vi "Rhythm Pattern Test.vi"() -> ()   [LabVIEW 2020]
uses:
  Rhythm Pattern VIs/Rhythm-Properties.ctl
  Rhythm Pattern VIs/Rhythm-Data.ctl
panel:
  out "Y-axis":dbl(slide) scale=-0.5..5.5
  out "Pattern":cluster{"X":dbl, "Y":dbl}[](graph)
  in  "Save Button":bool
  out "exit signal":bool
  out "Graph":dbl[](graph)
  out "finished":errorcluster
  in  "Play Button":bool
  in  "Refresh Button":bool
  in  "Quit Button":bool
  in  "Frame size (s)":dbl=0.25
  in  "Sampling rate (Hz)":dbl=50000.0
  in  "Properties":T1={"Method"=enum."Interval", "Waveform"=enum."Noise", "Time"={"Ramp (ms)"=5.0, "Duration (ms)"=25.0, "Interval (ms)"=400.0}, "Expr"="50:50:300", "Pattern"={"# rand"=5.0, "reg fraction"=1.0, "Rcyc"=5, "pattern"=enum."RAND-REG", "Lsignal (cyc)"={"Min"=12, "Max"=12}, "Trans (cyc)"={"Min"=4, "Max"=5}}}
  in  "Stop Button":bool
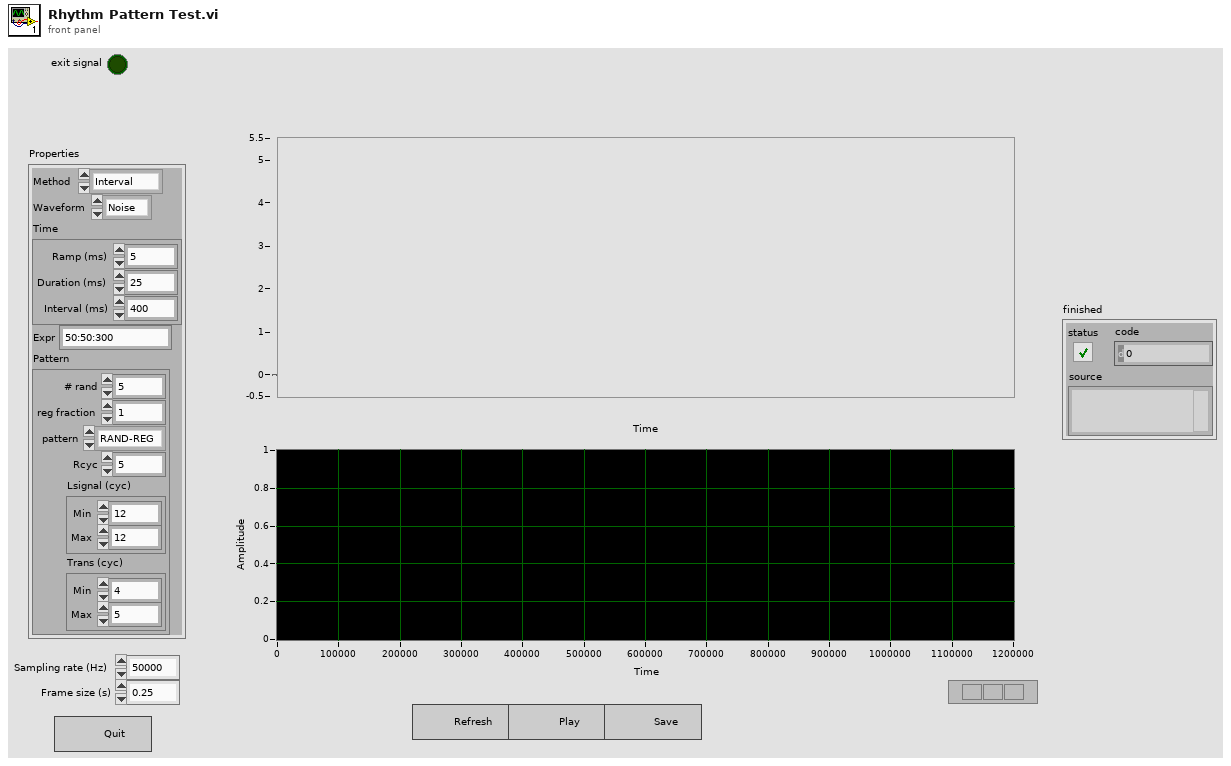
[diagram p1: front panel]
types:
  T1 = typedef "Rhythm-Properties.ctl" = cluster{"Method":enum16{"Telegraph", "Interval"}, "Waveform":enum16{"Click", "Noise"}, "Time":cluster{"Ramp (ms)":dbl, "Duration (ms)":dbl, "Interval (ms)":dbl}, "Expr":string, "Pattern":cluster{"# rand":dbl, "reg fraction":dbl, "Rcyc":i32, "pattern":enum16{"RAND-REG", "REG-RAND", "RAND", "REG", "STEP", "CF"}, "Lsignal (cyc)":cluster{"Min":i32, "Max":i32}, "Trans (cyc)":cluster{"Min":i32, "Max":i32}}}
  T2 = typedef "Rhythm-Data.ctl" = cluster{"Values":dbl[], "Gate":dbl[], "Rep":i32, "PhaseIndex":i32, "transition":i32, "nrepeat":i32, "Method":enum16{"Telegraph", "Interval"}, "Fs":dbl, "Time":cluster{"Ramp (ms)":dbl, "Duration (ms)":dbl, "Interval (ms)":dbl}, "Waveform":enum16{"Click", "Noise"}}
  T3 = cluster{"Data":T2, "Sampling rate (Hz)":dbl, i32, "#frames":i32}
  T4 = enum8{"Enabled", "Disabled", "Disabled and Grayed Out"}
  T5 = typedef "Sound Output Task ID.ctl" = u32
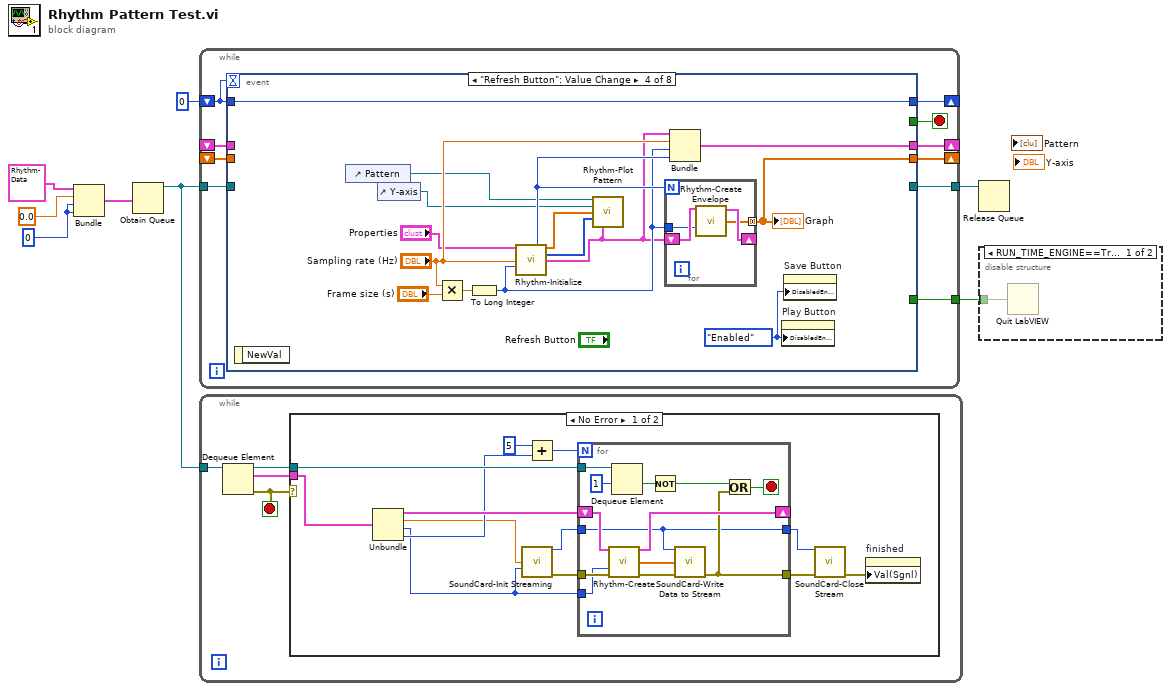
[diagram p0: block diagram]
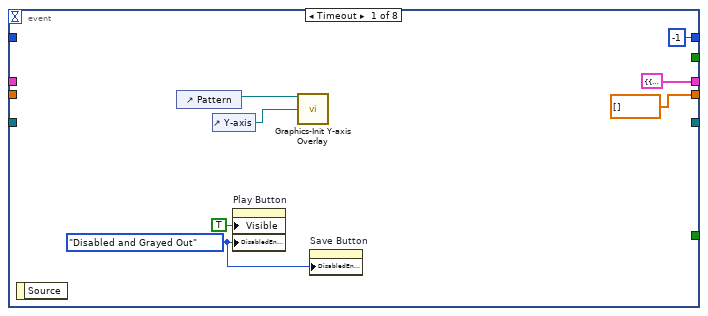
[diagram p4: hidden frame]
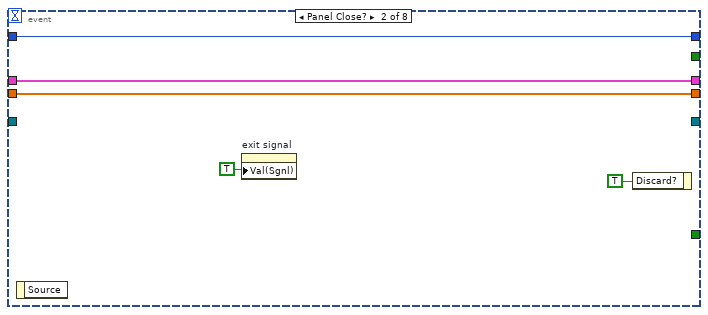
[diagram p5: hidden frame]
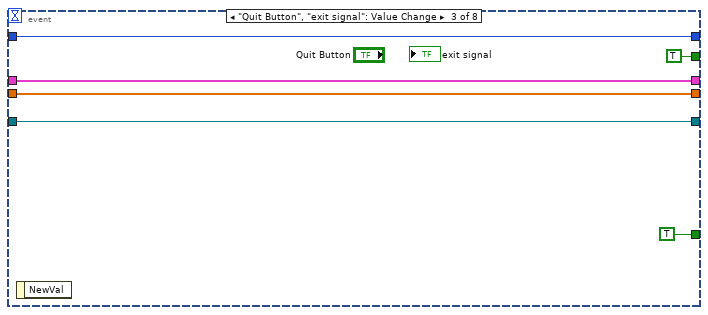
[diagram p6: hidden frame]
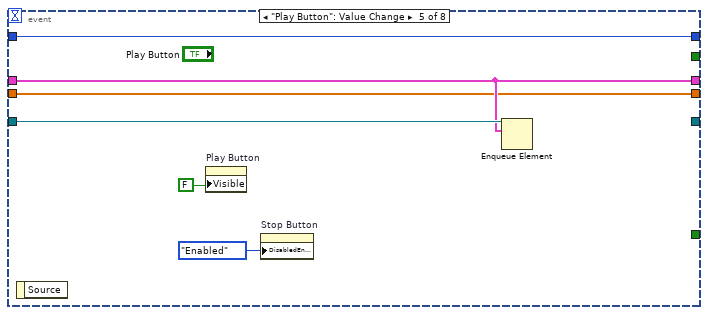
[diagram p7: hidden frame]
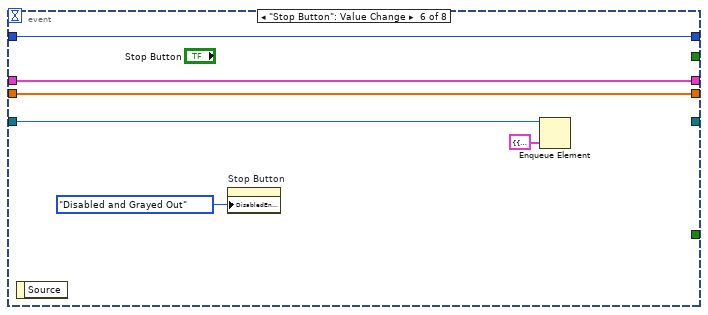
[diagram p8: hidden frame]
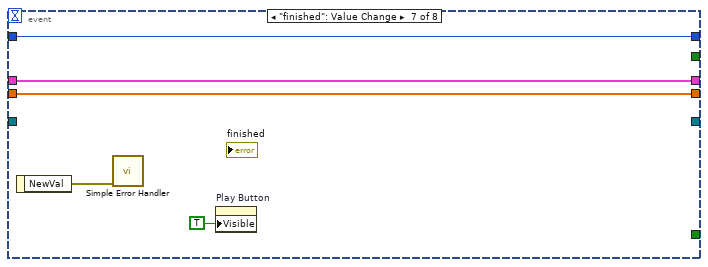
[diagram p9: hidden frame]
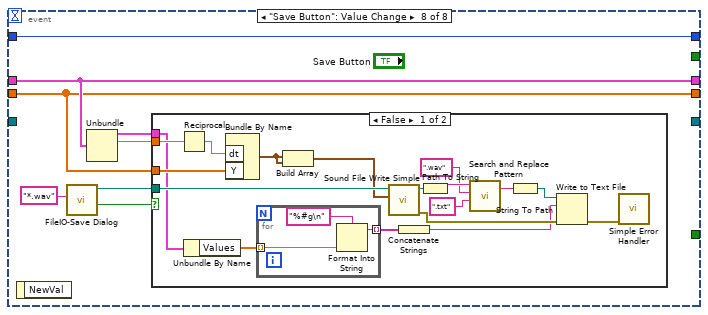
[diagram p10: hidden frame]
diagram:
  w2 = 0
  n1 = Bundle("Data"=T2 {"Values"=array[5000 elements], "Gate"=[8.0], "Rep"=0, "PhaseIndex"=5000, "transition"=0, "nrepeat"=0, "Method"=enum."Telegraph", "Fs"=0.0, "Time"={"Ramp (ms)"=0.0, "Duration (ms)"=0.0, "Interval (ms)"=0.0}, "Waveform"=enum."Click"}, 0.0, w2, w2) -> (w5:cluster{"Data":T2, dbl, i32, i32})  [unwired: 1 in]
  n2 = Obtain Queue(element data type=w5) -> (queue out=w6:refnum<queue>)  [unwired: 4 in, 2 out]
  n3 = while {
    shift-right: [w16] -> _
    shift-left: 0 -> [w17]
    tunnel: w6 -> [w15]
    tunnel: [w14] -> w7
    tunnel: [w13] -> w1
    shift-right: [w12] -> _
    shift-left: _ -> [w11]
    shift-right: [w10] -> _
    shift-left: _ -> [w9]
    stop <- w18 stop-if-true
    n4 = event shown="[3] \"Refresh Button\": Value Change" {
      selector: _ -> [_ _ _ _ _ _ _ _]
      dyn-events: _ -> [_ _ _ _ _ _ _ _]
      timeout: w17 -> [_ _ _ _ _ _ _ _]
      tunnel: [_ _ TRUE _ _ _ _ _] -> w18
      tunnel: w17 -> [_ w30 w35 w51 w61 w67 w72 w80]
      tunnel: [-1 w30 w35 w51 w61 w67 w72 w80] -> w16
      tunnel: w15 -> [_ _ w34 _ w58 w66 _ _]
      tunnel: [_ _ w34 _ _ _ _ _] -> w14
      tunnel: [_ _ TRUE _ _ _ _ _] -> w13
      tunnel: [T3 {"Data"={"Values"=[], "Gate"=[], "Rep"=0, "PhaseIndex"=0, "transition"=0, "nrepeat"=0, "Method"=enum."Telegraph", "Fs"=0.0, "Time"={"Ramp (ms)"=0.0, "Duration (ms)"=0.0, "Interval (ms)"=0.0}, "Waveform"=enum."Click"}, "Sampling rate (Hz)"=0.0, 0, "#frames"=0} w27 w32 w45 w57 w64 w69 w76] -> w12
      tunnel: w11 -> [_ w27 w32 _ w57 w64 w69 w76]
      tunnel: [dbl[] [] ("Y") w26 w31 w44 w56 w63 w68 w74] -> w10
      tunnel: w9 -> [_ w26 w31 _ w56 w63 w68 w74]
      event Timeout {
        w23 = T4."Disabled and Grayed Out" ("Disabled")
        n5 = event-data() -> ()  [unwired: 1 in, 1 out]
        n6 = control-ref of="Pattern"() -> (w20:refnum<vi>)
        n7 = control-ref of="Y-axis"() -> (w19:refnum<vi>)
        n8 = property on="Play Button" class="Bool"("Visible"=TRUE, "DisabledEnum"=w23) -> ()  [unwired: 2 in, 2 out]
        n9 = call "Graphics-Init Y-axis Overlay.vi"("Ctl Refnum"=w20, "Y-axis slider"=w19) -> ()  [unwired: 13 in, 1 out]
        n10 = property on="Save Button" class="Bool"("DisabledEnum"=w23) -> ()  [unwired: 2 in, 2 out]
      }
      event Panel Close? {
        n11 = event-data() -> ()  [unwired: 1 in, 1 out]
        n12 = property on="exit signal" class="Bool (strict)"("Val(Sgnl)"=TRUE ("Value (Signaling)")) -> ()  [unwired: 2 in, 2 out]
        n13 = event-data("Discard?"=TRUE) -> ()  [unwired: 1 in, 1 out]
      }
      event "Quit Button", "exit signal": Value Change {
        n14 = event-data() -> ()  [unwired: 1 in, 1 out]
      }
      event "Refresh Button": Value Change {
        w43 = T4."Enabled" ("Disabled")
        n15 = event-data() -> ()  [unwired: 1 in, 1 out]
        n16 = control-ref of="Pattern"() -> (w41:refnum<vi>)
        n17 = control-ref of="Y-axis"() -> (w40:refnum<vi>)
        n18 = Multiply(x="Sampling rate (Hz)", y="Frame size (s)") -> (x*y=w50:dbl)
        n19 = To Long Integer(number=w50) -> (32bit integer=w46:i32)
        n20 = call "Rhythm-Initialize.vi"("Rhythm"="Properties", "Sampling rate (Hz)"="Sampling rate (Hz)", "Npts"=w46) -> ("#frames"=w47:i32, "Values"=w39:dbl[], "Mask"=w38:i32[], "Data"=w37:T2)  [unwired: 8 in, 1 out]
        n21 = call "Rhythm-Plot Pattern.vi"("Graph"=w41, "Y-axis slider"=w40, "Values"=w39, "Mask"=w38, "Data"=w37) -> ()  [unwired: 10 in, 1 out]
        n22 = for {
          N: w47 -> [_]
          tunnel: w46 -> [w52]
          shift-right: [w54] -> _
          shift-left: w37 -> [w55]
          tunnel: [w53] -> w44 mode=concatenating
          n23 = call "Rhythm-Create Envelope.vi"("Data in"=w55, "Npts"=w52) -> ("Data out"=w54:T2, "Y"=w53:dbl[])  [unwired: 11 in, 1 out]
        }
        "Graph" <- w44
        n24 = Bundle("Data"=w37, "Sampling rate (Hz)"="Sampling rate (Hz)", w46, "#frames"=w47) -> (w45:T3)  [unwired: 1 in]
        n25 = property on="Play Button" class="Bool"("DisabledEnum"=w43) -> ()  [unwired: 2 in, 2 out]
        n26 = property on="Save Button" class="Bool"("DisabledEnum"=w43) -> ()  [unwired: 2 in, 2 out]
      }
      event "Play Button": Value Change {
        n27 = event-data() -> ()  [unwired: 1 in, 1 out]
        n28 = property on="Play Button" class="Bool"("Visible"=FALSE) -> ()  [unwired: 2 in, 2 out]
        n29 = property on="Stop Button" class="Bool"("DisabledEnum"=T4."Enabled" ("Disabled")) -> ()  [unwired: 2 in, 2 out]
        n30 = Enqueue Element(queue=w58, element=w57) -> ()  [unwired: 2 in, 3 out]
      }
      event "Stop Button": Value Change {
        n31 = event-data() -> ()  [unwired: 1 in, 1 out]
        n32 = property on="Stop Button" class="Bool"("DisabledEnum"=T4."Disabled and Grayed Out" ("Disabled")) -> ()  [unwired: 2 in, 2 out]
        n33 = Enqueue Element(queue=w66, element=cluster{"Data":T2, dbl, i32, i32} {"Data"={"Values"=[], "Gate"=[], "Rep"=0, "PhaseIndex"=0, "transition"=0, "nrepeat"=0, "Method"=enum."Telegraph", "Fs"=0.0, "Time"={"Ramp (ms)"=0.0, "Duration (ms)"=0.0, "Interval (ms)"=0.0}, "Waveform"=enum."Click"}, 0.0, 0, 0}) -> ()  [unwired: 2 in, 3 out]
      }
      event "finished": Value Change {
        n34 = event-data() -> ("NewVal"=w71:errorcluster)  [unwired: 1 in]
        n35 = call <vilib>:"Simple Error Handler.vi"("error in (no error)"=w71) -> ()  [unwired: 4 in, 5 out]
        n36 = property on="Play Button" class="Bool"("Visible"=TRUE) -> ()  [unwired: 2 in, 2 out]
      }
      event "Save Button": Value Change {
        n37 = event-data() -> ()  [unwired: 1 in, 1 out]
        n38 = call "FileIO-Save Dialog.vi"("pattern (all files)"="*.wav") -> ("cancelled"=w78:bool, "selected path"=w77:path)  [unwired: 8 in, 1 out]
        n39 = Unbundle(w76) -> ("Data"=w73:T2, "Sampling rate (Hz)"=w75:dbl)  [unwired: 2 out]
        n40 = case shown="False" w78 {
          tunnel: w77 -> [w98 _]
          tunnel: w75 -> [w97 _]
          tunnel: w74 -> [w95 _]
          tunnel: w73 -> [w92 _]
          frame False {
            n41 = Reciprocal(x=w97) -> (1/x=w96:dbl)
            n42 = Unbundle By Name(w92) -> ("Values"=w91:dbl[])
            n43 = Bundle By Name("dt"=w96, "Y"=w95) -> (w93:waveform(dbl))  [unwired: 1 in]
            n44 = for {
              tunnel: w91 -> [w99] mode=indexing
              tunnel: [w101] -> w82 mode=indexing
              n45 = Format Into String(format string="%#g\n", w99) -> (resulting string=w101:string)  [unwired: 2 in, 1 out]
            }
            n46 = Build Array(w93, w93) -> (w94:waveform(dbl)[])
            n47 = call <vilib>:"Sound File Write Simple.vi"("data"=w94, "path"=w98) -> ("error out"=w85:errorcluster, "path out"=w90:path)  [unwired: 8 in]
            n48 = Concatenate Strings(w82) -> (w81:string)
            n49 = Path To String(path=w90) -> (string=w89:string)
            n50 = call <vilib>:"Search and Replace Pattern.vi"("string"=w89, "regular expression (\"\")"=".wav" ("regular expression (\"\")"), "replace string (\"\")"=".txt" ("replace string (\"\")")) -> ("result string"=w86:string)  [unwired: 2 in, 1 out]
            n51 = String To Path(string=w86) -> (path=w84:path)
            n52 = Write to Text File(file (use dialog)=w84, text=w81, error in=w85) -> (error out=w83:errorcluster)  [unwired: 1 in, 2 out]
            n53 = call <vilib>:"Simple Error Handler.vi"("error in (no error)"=w83) -> ()  [unwired: 4 in, 5 out]
          }
          frame True {
          }
        }
      }
    }
  }
  n54 = while {
    tunnel: w6 -> [w105]
    stop <- w102 stop-if-true
    n55 = Dequeue Element(queue=w105) -> (queue out=w103:refnum<queue>, element=w104:cluster{"Data":T2, dbl, i32, i32}, error out=w102:errorcluster)  [unwired: 2 in, 1 out]
    n56 = case shown="No Error" w102 {
      tunnel: w104 -> [w117 _]
      tunnel: w103 -> [w118 _]
      frame No Error {
        n57 = Unbundle(w117) -> ("Data"=w109:T2, w106:dbl, w107:i32, w108:i32)
        n58 = call "SoundCard-Init Streaming.vi"("sample rate (S/s)"=w106, "Npts"=w107) -> ("task ID"=w115:T5, "error out"=w116:errorcluster)  [unwired: 12 in]
        n59 = Add(x=5, y=w108) -> (x+y=w111:i32)
        n60 = for {
          N: w111 -> [_]
          tunnel: w118 -> [w131]
          tunnel: w116 -> [w126]
          tunnel: [w122] -> w114
          shift-right: [w124] -> _
          shift-left: w109 -> [w125]
          tunnel: w107 -> [w119]
          tunnel: w115 -> [w121]
          tunnel: [w121] -> w112
          stop <- w127 stop-if-true
          n61 = call "Rhythm-Create.vi"("Data in"=w125, "Npts"=w119, "error in (no error)"=w126) -> ("Data out"=w124:T2, "Y"=w120:dbl[], "error out"=w123:errorcluster)  [unwired: 10 in]
          n62 = Dequeue Element(queue=w131, timeout in ms (-1)=1) -> (timed out?=w129:bool)  [unwired: 1 in, 3 out]
          n63 = Not(x=w129) -> (.not. x?=w128:bool)
          n64 = call "SoundCard-Write Data to Stream.vi"("task ID"=w121, "Array"=w120, "error in (no error)"=w123) -> ("error out"=w122:errorcluster)  [unwired: 11 in, 1 out]
          n65 = Or(x=w128, y=w122) -> (x .or. y?=w127:bool)
        }
        n66 = call "SoundCard-Close Stream.vi"("task ID"=w112, "error in (no error)"=w114) -> ("error out"=w113:errorcluster)  [unwired: 13 in]
        n67 = property on="finished" class="Clust (strict)"("Val(Sgnl)"=w113) -> ()  [unwired: 2 in, 2 out]
      }
      frame Error {
      }
    }
  }
  n68 = Release Queue(queue=w7) -> ()  [unwired: 2 in, 3 out]
  n69 = disable-structure shown="RUN_TIME_ENGINE==True" {
    disable-tunnel: w1 -> [w132 _]
    frame condition #0 {
      n70 = Quit LabVIEW(quit? (T)=w132) -> ()
    }
    frame condition #1 (active) {
    }
  }
